vi "Validate Configuration (Transfer).vi"(8 "error in (no error)":errorcluster, 11 "transfer configuration in":T1 {"channels"."string offset" format="%d bytes"}) -> (0 "error out":errorcluster, 3 "transfer configuration out":T1 {"channels"."string offset" format="%d bytes"})   [LabVIEW 2017, in "DSF Core.lvlib"]
uses:
  DSF Core.lvlib
  Typedefs/DSF Engine Transfer Configuration.ctl
  Typedefs/DSF Byte Order.ctl
  Typedefs/DSF Settings Info.ctl
  Typedefs/DSF Engine Channel Configuration.ctl
  Typedefs/DSF Data Type.ctl
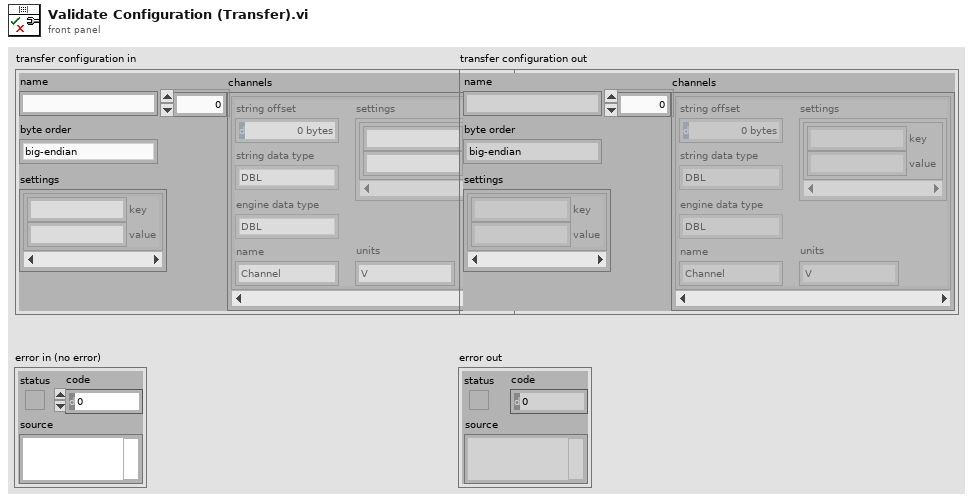
[diagram p1: front panel]
types:
  T1 = typedef "DSF Core.lvlib/DSF Engine Transfer Configuration.ctl" = cluster{"name":string, "byte order":T2, "settings":T3, "channels":T4[]}
  T2 = typedef "DSF Core.lvlib/DSF Byte Order.ctl" = enum8{"big-endian", "little-endian"}
  T3 = typedef "DSF Core.lvlib/DSF Settings Info.ctl" = cluster{"key":string, "value":string}[]
  T4 = typedef "DSF Core.lvlib/DSF Engine Channel Configuration.ctl" = cluster{"string offset":u64, "string data type":T5, "engine data type":T5, "name":string, "settings":T3, "units":string}
  T5 = typedef "DSF Core.lvlib/DSF Data Type.ctl" = enum8{"Bool", "SGL", "DBL", "I8", "I16", "I32", "I64", "U8", "U16", "U32", "U64"}
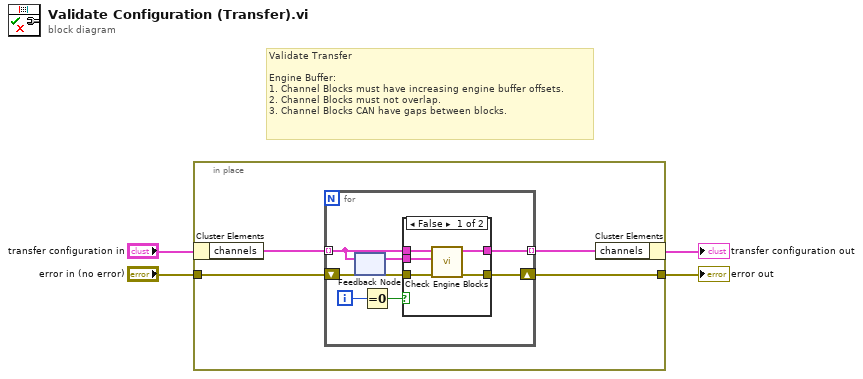
[diagram p0: block diagram]
diagram:
  # "Validate Transfer\n\nEngine Buffer:\n1. Channel Blocks must have increasing engine buffer offsets.\n2. Channel Blocks must not overlap.\n3. Channel Blocks CAN have gaps between blocks."
  n1 = in-place {
    in-place-border: [w8] -> w4
    in-place-border: "error in (no error)" -> [w7]
    n2 = in-place-cluster #1("transfer configuration in") -> ("channels"=w6:T4[])
    n3 = for {
      tunnel: w6 -> [w13] mode=indexing
      tunnel: [w11] -> w5 mode=indexing
      shift-right: [w10] -> w8
      shift-left: w7 -> [w9]
      i -> [w15]
      n4 = feedback #2() -> (w12:T4)  [unwired: 1 in]
      n5 = feedback-in #2(w13) -> ()
      n6 = Equal To 0?(x=w15) -> (x = 0?=w14:bool)
      n7 = case shown="False" w14 {
        tunnel: w13 -> [w17 w21]
        tunnel: [w17 w21] -> w11
        tunnel: w12 -> [w19 _]
        tunnel: [w16 w20] -> w10
        tunnel: w9 -> [w18 w20]
        frame False {
          n8 = call "Check Engine Blocks.vi"("error in (no error)"=w18, "previous channel block"=w19, "channel block"=w17) -> ("error out"=w16:errorcluster)  [unwired: 8 in]
        }
        frame True {
        }
      }
    }
    n9 = in-place-cluster #1("channels"=w5) -> (→"transfer configuration out":T1)
  }
  "error out" <- w4
